vi "CheckCollisions.vi"(8 "error in (no error)":errorcluster, 11 "Game Data":T2) -> (0 "error out":errorcluster, 3 "Next Cell Action":T1)   [LabVIEW 2020]
uses:
  TypeDef/game-data.ctl
  TypeDef/tiles-key.ctl
  TypeDef/direction.ctl
  TypeDef/next-cell-action.ctl
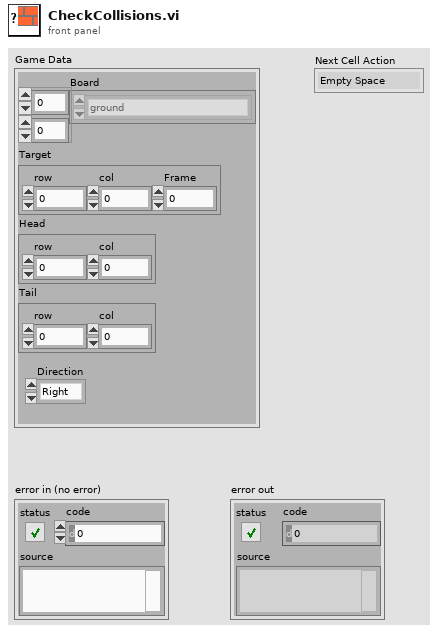
[diagram p1: front panel]
types:
  T1 = typedef "next-cell-action.ctl" = enum16{"Empty Space", "Target Captured", "Collision"}
  T2 = typedef "game-data.ctl" = cluster{"Board":T3[][], "Target":cluster{"row":i32, "col":i32, "Frame":i8}, "Head":cluster{"row":i32, "col":i32}, "Tail":cluster{"row":i32, "col":i32}, "Direction":T4}
  T3 = typedef "tiles-key.ctl" = enum16{"ground", "wall", "head (right)", "head (up)", "head (left)", "head (down)", "L-turn (right-up)", "L-turn (up-left)", "L-turn (left-down)", "L-turn (down-right)", "body (right)", "body (up)", "body (left)", "body (down)", "R-turn (right-down)", "R-turn (up-right)", "R-turn (left-up)", "R-turn (down-left)", "tail (right)", "tail (up)", "tail (left)", "tail (down)", "dead head (right)", "dead head (up)", "dead head (left)", "dead head (down)", "dead L-turn (right-up)", "dead L-turn (up-left)", "dead L-turn (left-down)", "dead L-turn (down-right)", "dead body (right)", "dead body (up)", "dead body (left)", "dead body (down)", "dead R-turn (right-down)", "dead R-turn (up-right)", "dead R-turn (left-up)", "dead R-turn (down-left)", "dead tail (right)", "dead tail (up)", "dead tail (left)", "dead tail (down)", "target red", "target blue", "target yellow", "target green"}
  T4 = typedef "direction.ctl" = enum16{"Right", "Up", "Left", "Down"}
  T5 = enum16{"Empty Space", "Target Captured", "Collision"}
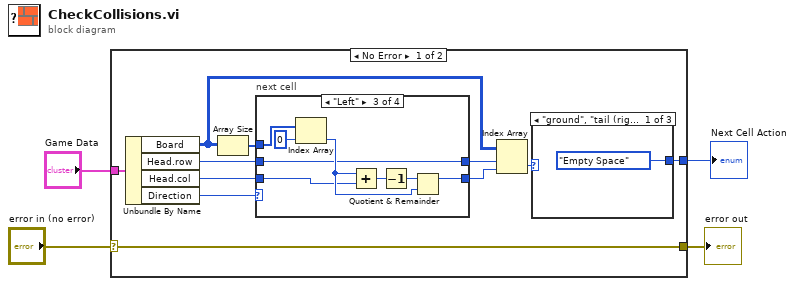
[diagram p0: block diagram]
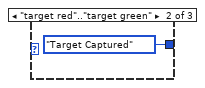
[diagram p2: hidden frame]
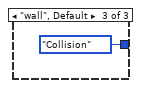
[diagram p3: hidden frame]
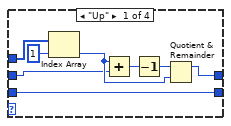
[diagram p4: hidden frame]
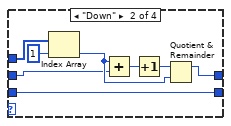
[diagram p5: hidden frame]
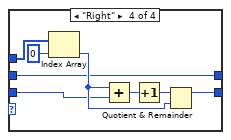
[diagram p6: hidden frame]
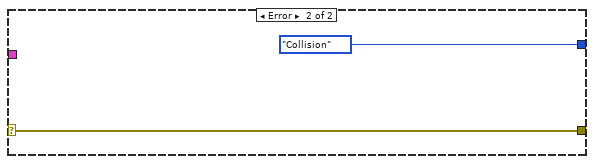
[diagram p7: hidden frame]
diagram:
  n1 = case shown="No Error" "error in (no error)" {
    selector: "error in (no error)" -> [w15 w52]
    tunnel: [w15 w52] -> w3
    tunnel: "Game Data" -> [w14 _]
    tunnel: [w5 T5."Collision" ("Enum")] -> w1
    frame No Error {
      n2 = Unbundle By Name(w14) -> ("Board"=w13:T3[][], "Head.row"=w11:i32, "Head.col"=w10:i32, "Direction"=w12:T4)
      n3 = Array Size(array=w13) -> (size(s)=w9:i32[])
      n4 = case "next cell" shown="\"Left\"" w12 {
        tunnel: w11 -> [w21 w29 w35 w43]
        tunnel: w10 -> [w20 w28 w37 w45]
        tunnel: w9 -> [w26 w34 w42 w50]
        tunnel: [w20 w28 w36 w44] -> w7
        tunnel: [w19 w27 w35 w43] -> w8
        frame "Up" {
          n5 = Index Array(array=w26, index=1) -> (element=w23:i32)
          n6 = Add(x=w23, y=w21) -> (x+y=w24:i32)
          n7 = Decrement(x=w24) -> (x-1=w22:i32)
          n8 = Quotient & Remainder(x=w22, y=w23) -> (x-y*floor(x/y)=w19:i32)  [unwired: 1 out]
        }
        frame "Down" {
          n9 = Index Array(array=w34, index=1) -> (element=w31:i32)
          n10 = Add(x=w31, y=w29) -> (x+y=w32:i32)
          n11 = Increment(x=w32) -> (x+1=w30:i32)
          n12 = Quotient & Remainder(x=w30, y=w31) -> (x-y*floor(x/y)=w27:i32)  [unwired: 1 out]
        }
        frame "Left" {
          n13 = Index Array(array=w42, index=0) -> (element=w39:i32)
          n14 = Add(x=w39, y=w37) -> (x+y=w40:i32)
          n15 = Decrement(x=w40) -> (x-1=w38:i32)
          n16 = Quotient & Remainder(x=w38, y=w39) -> (x-y*floor(x/y)=w36:i32)  [unwired: 1 out]
        }
        frame "Right" {
          n17 = Index Array(array=w50, index=0) -> (element=w47:i32)
          n18 = Add(x=w47, y=w45) -> (x+y=w48:i32)
          n19 = Increment(x=w48) -> (x+1=w46:i32)
          n20 = Quotient & Remainder(x=w46, y=w47) -> (x-y*floor(x/y)=w44:i32)  [unwired: 1 out]
        }
      }
      n21 = Index Array(array=w13, index (row)=w8, index (col)=w7) -> (element=w6:T3)
      n22 = case shown="\"ground\", \"tail (right)\"..\"tail (down)\"" w6 {
        tunnel: [T5."Empty Space" ("Enum") T5."Target Captured" ("Enum") T5."Collision" ("Enum")] -> w5
        frame "ground", "tail (right)".."tail (down)" {
        }
        frame "target red".."target green" {
        }
        frame "wall", Default {
        }
      }
    }
    frame Error {
    }
  }
  "error out" <- w3
  "Next Cell Action" <- w1
